vi "SetsystimeCMD.vi"() -> ()   [LabVIEW 2015]
panel:
  out "standard output":string caption="标准输出"
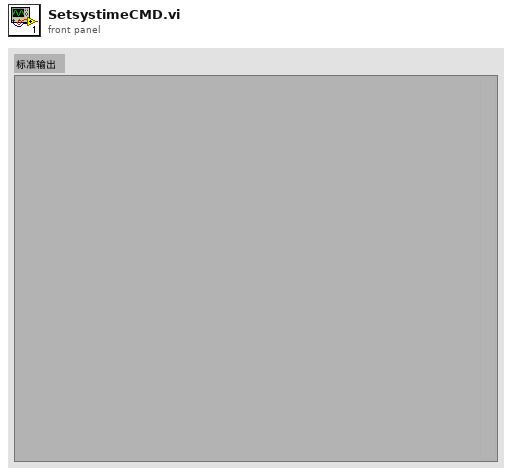
[diagram p1: front panel]
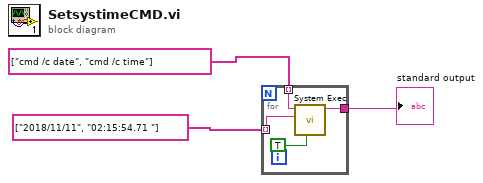
[diagram p0: block diagram]
diagram:
  n1 = for {
    tunnel: string[] ["2018/11/11", "02:15:54.71 "] ("standard input") -> [w7] mode=indexing
    tunnel: string[] ["cmd /c date", "cmd /c time"] ("command line") -> [w5] mode=indexing
    tunnel: [w4] -> w1
    n2 = call <vilib>:"System Exec.vi"("run minimized? (F)"=TRUE, "standard input"=w7, "command line"=w5) -> ("standard output"=w4:string)  [unwired: 5 in, 3 out]
  }
  "standard output" <- w1
